vi "Constants.vi"() -> ()   [LabVIEW 2014, in "ParametericRoutines.lvlib"]
uses:
  ParametericRoutines.lvlib
panel:
  in  "App.Sufix":string=".AppVersion"
  in  "Boot.Sufix":string=".BootVersion"
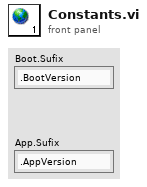
[diagram p1: front panel]
diagram:
